vi "AnotherClass_GetAttributes.vi"(0 "reference in":refnum<class "AnotherClass.lvclass">, 5 "error in (no error)":errorcluster) -> (14 "reference out":refnum<class "AnotherClass.lvclass">, 16 "Attributes":T1 {"Attribute1" format="%.2f"}, 17 "Attributes locked?":bool, 19 "error out":errorcluster)   [LabVIEW 2016, in "AnotherClass.lvclass"]
doc: "Returns the attributes of this class or subclass object.\n\nIf the object is currently locked for modification, 'Attibutes locked?' will return TRUE."
uses:
  <vilib>/addons/GOOPUtility/_Demo/GOOPUtil_Demo/AnotherClass_class/AnotherClass.lvclass
  <vilib>/addons/GOOPUtility/_Demo/GOOPUtil_Demo/AnotherClass_class/protected/ObjectAttributes.ctl
  <vilib>/addons/_goop3.llb/3GOOPStates.ctl
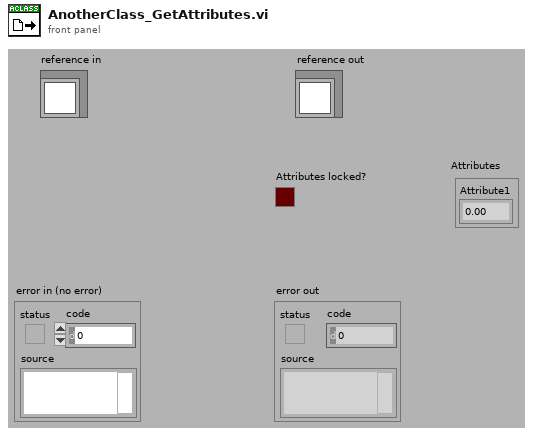
[diagram p1: front panel]
types:
  T1 = typedef "AnotherClass.lvclass/ObjectAttributes.ctl" = cluster{"Attribute1":dbl}
  T2 = typedef "3GOOPStates.ctl" = enum16{"Set", "Get", "New", "Delete", "Clear", "Test and get", "Unlock data", "Information", "Look up existing", "New or look up existing", "Test and get shared", "Get shared", "Set shared", "Unlock shared", "Find dynamic method", "Register dynamic method", "Preload dynamic method", "Probe", "Cast to more generic", "Cast to more specific"}
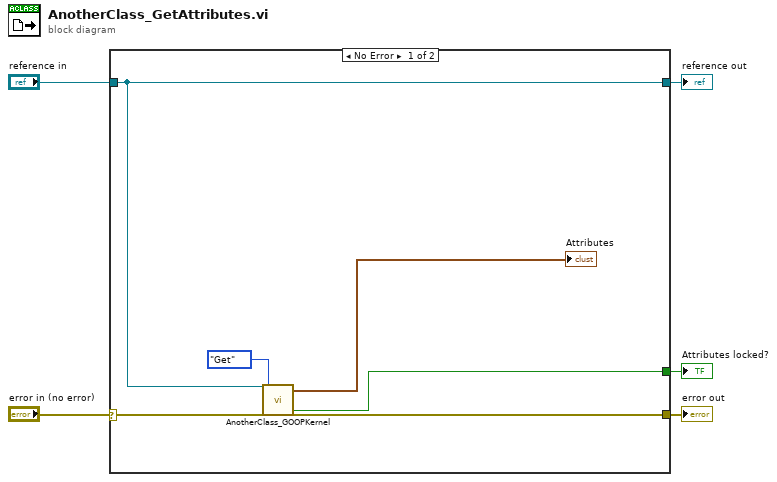
[diagram p0: block diagram]
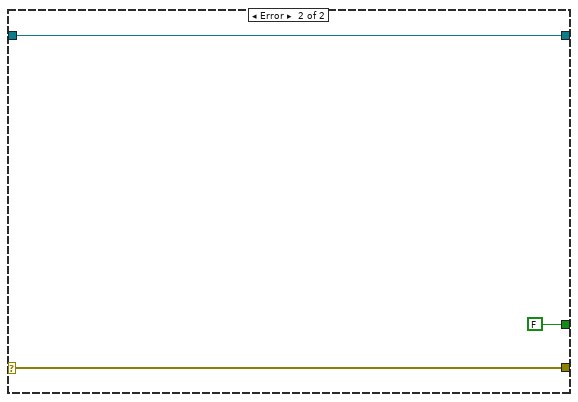
[diagram p2: hidden frame]
diagram:
  n1 = case shown="No Error" "error in (no error)" {
    selector: "error in (no error)" -> [w11 w13]
    tunnel: [w6 w14] -> w5
    tunnel: [w10 w13] -> w4
    tunnel: "reference in" -> [w6 w14]
    tunnel: [w9 FALSE ("Data locked?")] -> w1
    frame No Error {
      n2 = call <vilib>:"AnotherClass_GOOPKernel.vi"("Ref in"=w6, "error in (no error)"=w11, "Action"=3GOOPStates."Get") -> ("Data out"=→"Attributes":T1, "Data locked?"=w9:bool, "error out"=w10:errorcluster)  [unwired: 14 in, 8 out]
    }
    frame Error {
    }
  }
  "error out" <- w4
  "reference out" <- w5
  "Attributes locked?" <- w1
